vi "Actor Core.vi"(8 "error in":errorcluster, 11 "Actor with Nesteds in":refnum<class "Actor with Nesteds.lvclass">) -> (0 "error out":errorcluster, 3 "Actor out":refnum<class "Actor.lvclass">)   [LabVIEW 2020, in "Actor with Nesteds.lvlib" / "Actor with Nesteds.lvclass"]
doc: "<p>(<strong>Filename</strong>: <span class=\"dnl\">Actor Framework.lvlib:Actor.lvclass:Actor Core.vi</span>)</p>\n<p>Receives messages to the actor, reacts to them, and initiates any error handling that may shut the actor down.</p>\n<p>Descendant classes may override this VI to append parallel tasks for the actor to complete while it handles messages. Overrides use the <a href=\"nihelplauncher://docs/csh?context=lvcore_glang_udclass\">Call Parent Class Method</a> node.</p>"
uses:
  Actor with Nesteds.lvclass
  C:/Users/J63553/Projects/_LabVIEW Community/actor-framework/Core/ActorFramework/Actor/Actor.lvclass
  Core/ActorFramework/Actor/Actor.lvclass
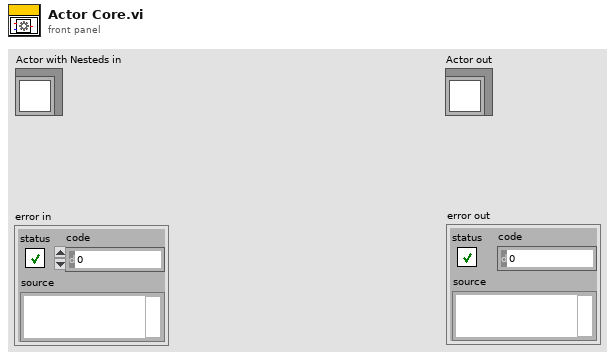
[diagram p1: front panel]
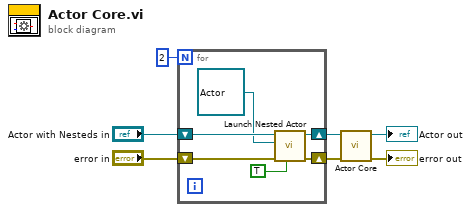
[diagram p0: block diagram]
diagram:
  n1 = for {
    N: 2 -> [_]
    shift-right: [w12] -> w4
    shift-left: "error in" -> [w13]
    shift-right: [w11] -> w3
    shift-left: "Actor with Nesteds in" -> [w10]
    n2 = call "Launch Nested Actor.vi"("Open Actor Core front panel? (F)"=TRUE, "error in (no error)"=w13, "Nested Actor"=refnum<class "Actor.lvclass"> refnum ("Actor Framework:Actor"), "Caller Actor in"=w10) -> ("error out"=w12:errorcluster, "Caller Actor out"=w11:refnum<class "Actor with Nesteds.lvclass">)  [unwired: 5 in, 1 out]
  }
  n3 = call-parent "Actor Core.vi"("error in"=w4, "Actor in"=w3) -> ("error out"=→"error out":errorcluster, "Actor out"=→"Actor out":refnum<class "Actor.lvclass">)  [unwired: 8 in]
